vi "AFM_Litho_Plugin.IV.NewLockinAddress.vi"(8 "error in (no error)":errorcluster, 10 "NewLockinAddress":T1, 11 "AFM_Litho_Plugin.IV":refnum<class "AFM_Litho_Plugin.IV.lvclass">) -> (0 "error out":errorcluster, 3 "AFM_Litho_Plugin.IV out":refnum<class "AFM_Litho_Plugin.IV.lvclass">)   [LabVIEW 2019, in "AFM_Litho_Plugin.IV.lvclass"]
doc: "---------------------------------------------------------------\nJKI State Machine Objects™\nhttp://jki.net/state-machine-objects/\nCopyright (C) 2005-2015, JKI <info@jki.net>\nALL RIGHTS RESERVEDJKI State Machine Objects (SMO) 1.0.0.4\nJKI - JKI\nCopyright (c) 2015, JKI"
uses:
  AFM_Litho_Plugin.IV.lvclass
  Typedefs/PrivateEvents--AFM_Litho_Plugin.IV.NewLockinAddress.ctl
  AFM_Litho_Plugin.IV.lvclass/AFM_Litho_Plugin.IV.ctl
panel:
  # "For instructions on how to use the JKI State Machine Objects, examples and video tutorials, visit:\nhttp://jki.net/state-machine-objects/\n\nJKI State Machine Objects™\nhttp://jki.net/state-machine-objects/\nCopyright (C) 2005-2015, JKI <info@jki.net>\nALL RIGHTS RESERVED"
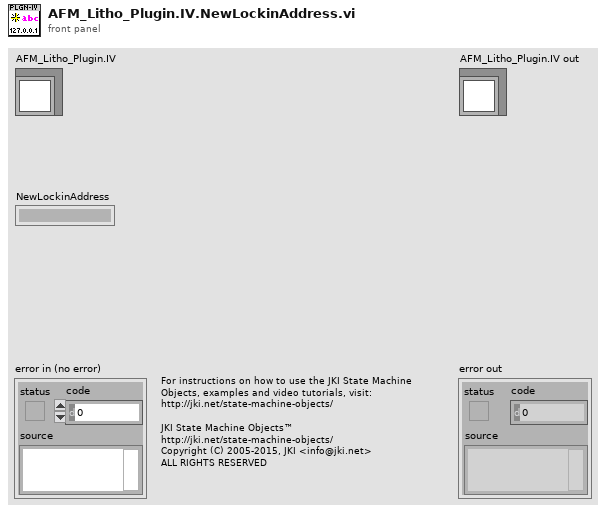
[diagram p1: front panel]
types:
  T1 = typedef "AFM_Litho_Plugin.IV.lvclass/PrivateEvents--AFM_Litho_Plugin.IV.NewLockinAddress.ctl" = string
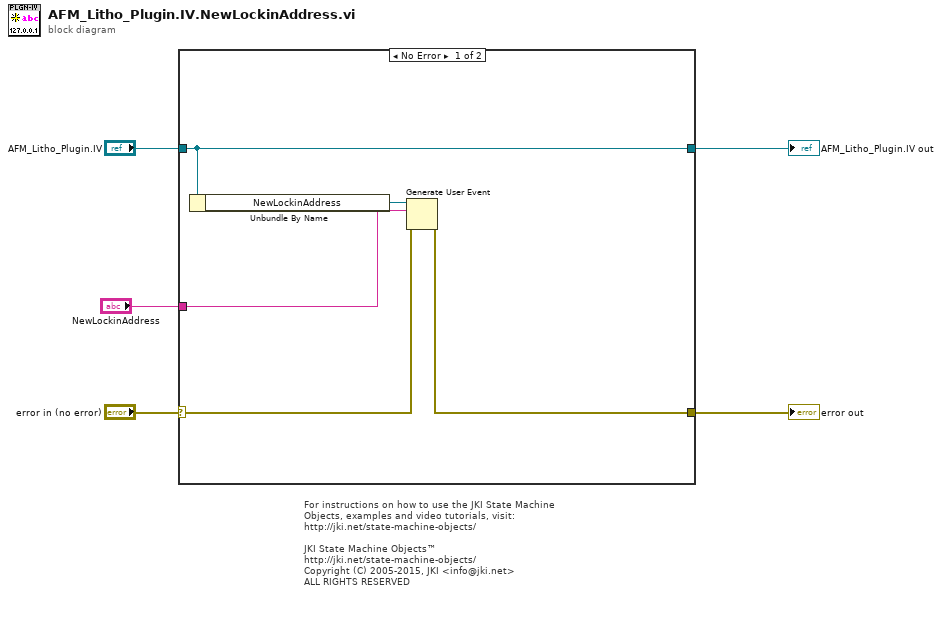
[diagram p0: block diagram]
diagram:
  # "For instructions on how to use the JKI State Machine Objects, examples and video tutorials, visit:\nhttp://jki.net/state-machine-objects/\n\nJKI State Machine Objects™\nhttp://jki.net/state-machine-objects/\nCopyright (C) 2005-2015, JKI <info@jki.net>\nALL RIGHTS RESERVED"
  n1 = case shown="No Error" "error in (no error)" {
    selector: "error in (no error)" -> [w10 w12]
    tunnel: [w7 w12] -> w4
    tunnel: [w6 w11] -> w5
    tunnel: "AFM_Litho_Plugin.IV" -> [w6 w11]
    tunnel: "NewLockinAddress" -> [w9 _]
    frame No Error {
      n2 = Unbundle By Name(w6) -> ("NewLockinAddress"=w8:refnum<user-event>)
      n3 = Generate User Event(user event=w8, event data cluster=w9, error in=w10) -> (error out=w7:errorcluster)  [unwired: 1 in, 1 out]
    }
    frame Error {
    }
  }
  "error out" <- w4
  "AFM_Litho_Plugin.IV out" <- w5
